vi "conv.vi"() -> ()   [LabVIEW 2013]
uses:
  <vilib>/Analysis/2dsp.llb/1D Convolution (DBL).vi
  <vilib>/Analysis/NI_AALPro.lvlib
panel:
  out "大小":i32
  out "波形图":dbl[][](graph)
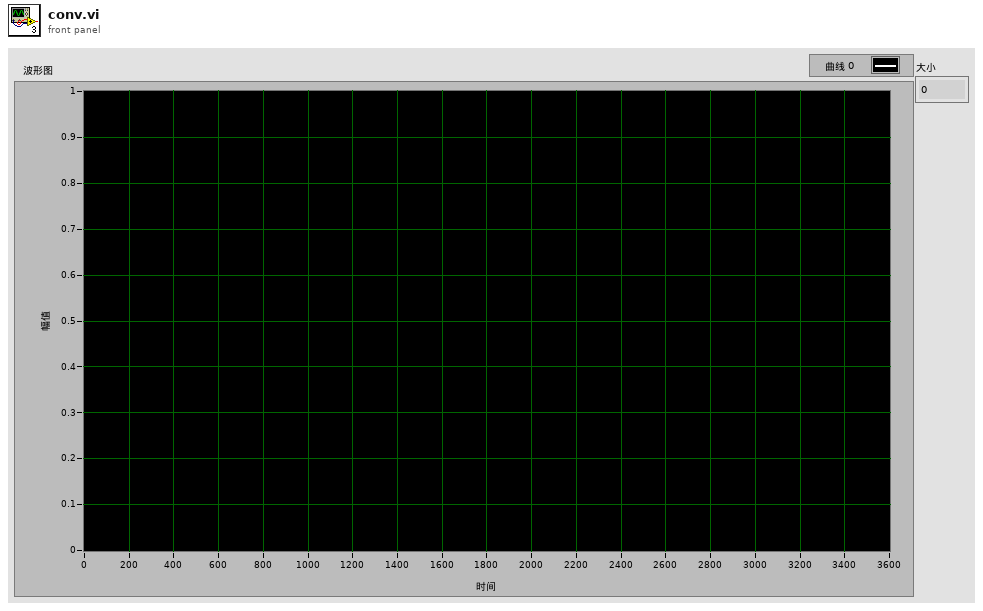
[diagram p1: front panel]
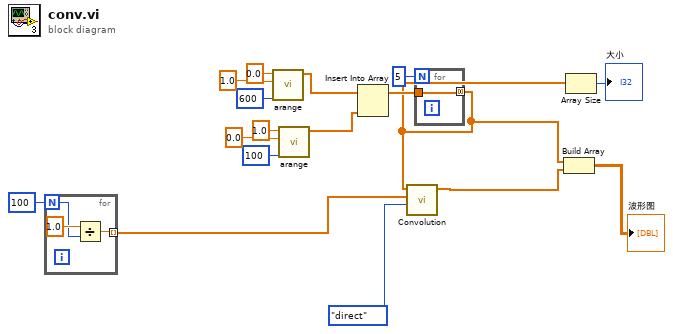
[diagram p0: block diagram]
diagram:
  n1 = for {
    N: 100 -> [w19]
    tunnel: [w18] -> w12 mode=indexing
    n2 = Divide(x=1.0, y=w19) -> (x/y=w18:dbl)
  }
  n3 = call "arange.vi"("Number of pixels"=600, "end"=1.0, "begin"=0.0) -> ("数组"=w8:dbl[])  [unwired: 8 in]
  n4 = call "arange.vi"("Number of pixels"=100, "end"=0.0, "begin"=1.0) -> ("数组"=w7:dbl[])  [unwired: 8 in]
  n5 = Insert Into Array(array=w8, new element=w7) -> (w5:dbl[])  [unwired: 1 in]
  n6 = for {
    N: 5 -> [_]
    tunnel: [w21] -> w3 mode=concatenating
    tunnel: w5 -> [w21]
  }
  n7 = call-poly <vilib>:"Convolution.vi"("algorithm"=enum32{"direct", "frequency domain"}."direct", "Y"=w12, "X"=w3) -> ("X * Y"=w2:dbl[])  [unwired: 7 in, 1 out]
  n8 = Build Array(w3, w2) -> (→"波形图":dbl[][])
  n9 = Array Size(array=w3) -> (size(s)=→"大小":i32)
